vi "VarianttoQueueData.vi"(8 "Error In":errorcluster, 10 "TimedOut":bool, 11 "Variant":variant) -> (0 "Error Out":errorcluster, 1 "Class":refnum<class "SensorBase.lvclass">, 2 "Message Data":variant, 3 "Message":string)   [LabVIEW 2018, in "SensorPlugins.lvlib"]
uses:
  SensorPlugins.lvlib
  SensorBaseClass/SensorBase.lvclass
  clMessage.ctl
panel:
  out "timed out?":bool
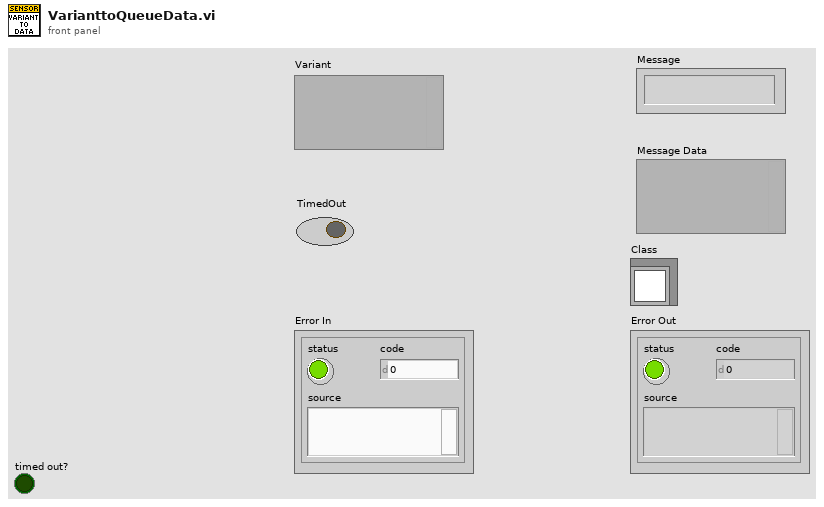
[diagram p1: front panel]
types:
  T1 = typedef "SensorPlugins.lvlib/clMessage.ctl" = cluster{"Message":string, "Message Data":variant, "Class":refnum<class "SensorBase.lvclass">}
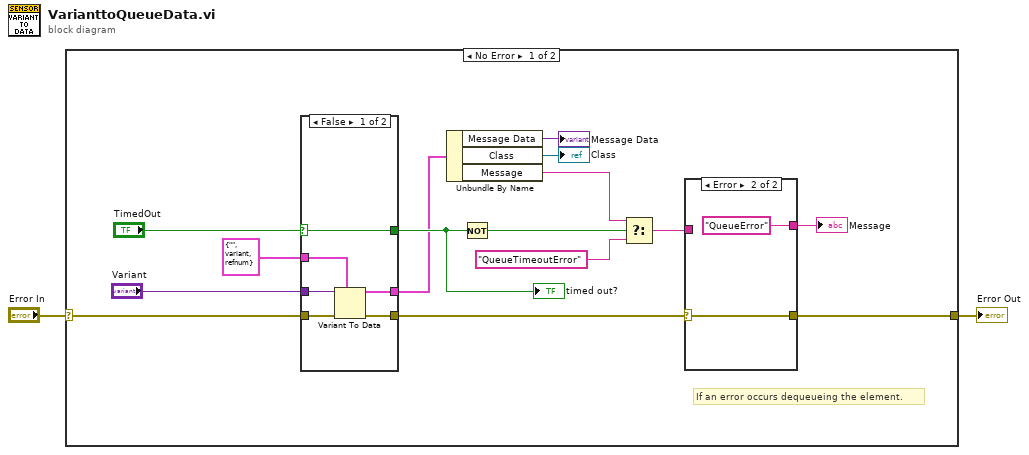
[diagram p0: block diagram]
diagram:
  n1 = case shown="No Error" "Error In" {
    selector: "Error In" -> [w6 w31]
    tunnel: [w5 w31] -> w1
    frame No Error {
      # "If an error occurs dequeueing the element."
      n2 = case shown="False" "TimedOut" {
        selector: "TimedOut" -> [w23 w26]
        tunnel: [w23 w26] -> w10
        tunnel: "Variant" -> [w22 _]
        tunnel: w6 -> [w21 w25]
        tunnel: [w20 w25] -> w9
        tunnel: [w19 w24] -> w7
        tunnel: T1 {"Message"="", "Message Data"=variant, "Class"=refnum} ("clMessage") -> [w18 w24]
        frame False {
          n3 = Variant To Data(error in=w21, type=w18, Variant=w22) -> (data=w19:T1, error out=w20:errorcluster)
        }
        frame True {
        }
      }
      "timed out?" <- w10
      n4 = Unbundle By Name(w7) -> ("Message Data"=→"Message Data":variant, "Class"=→"Class":refnum<class "SensorBase.lvclass">, "Message"=w14:string)
      n5 = Not(x=w10) -> (.not. x?=w13:bool)
      n6 = Select(t=w14, s=w13, f="QueueTimeoutError" ("Message")) -> (s? t:f=w12:string)
      n7 = case shown="Error" w9 {
        selector: w9 -> [w27 w29]
        tunnel: w12 -> [w28 _]
        tunnel: [w28 "QueueError" ("Message")] -> w15
        tunnel: [w27 w29] -> w5
        frame No Error {
        }
        frame Error {
        }
      }
      "Message" <- w15
    }
    frame Error {
    }
  }
  "Error Out" <- w1
